vi "Core Iterate.vi"(8 "error in (no error)":errorcluster, 11 "Function in":refnum<class "Function.lvclass">) -> (0 "error out":errorcluster, 3 "Function out":refnum<class "Function.lvclass">)   [LabVIEW 2016, in "Function Actor.lvlib" / "Function.lvclass"]
uses:
  <userlib>/Common Components/Function Actor/Function.lvclass
  C:/Program Files (x86)/National Instruments/LabVIEW 2016/vi.lib/ActorFramework/Actor/Actor.lvclass
  <vilib>/ActorFramework/Actor/Actor.lvclass/Actor.ctl
  <vilib>/ActorFramework/Message Enqueuer/Message Enqueuer.lvclass/Message Enqueuer.ctl
  <userlib>/Common Components/Function Actor/Function.lvclass/Function.ctl
  <userlib>/Common Components/Function Actor/Accessors/Read polling interval (ms).vi
  <vilib>/ActorFramework/Message Enqueuer/Init from Existing Queue.vi
  <vilib>/ActorFramework/Message Enqueuer/Enqueue.vi
  <userlib>/Common Components/Function Messages/Monitoring Msg/Monitoring Msg.lvclass
  C:/Program Files (x86)/National Instruments/LabVIEW 2016/vi.lib/ActorFramework/Message/Message.lvclass
  <userlib>/Common Components/Function Messages/Updating Msg/Updating Msg.lvclass
  <userlib>/Common Components/Function Messages/Dec No of Core Iter Msg/Wait till Interval Msg.lvclass
  <userlib>/Common Components/Function Actor/Messages/Acquire Msg/Core Iterate Msg.lvclass
  <vilib>/ActorFramework/Message Priority Queue/Priority Enqueue.vi
  <vilib>/ActorFramework/Message Enqueuer/Message Enqueuer.lvclass
  <vilib>/ActorFramework/Actor/Actor.lvclass
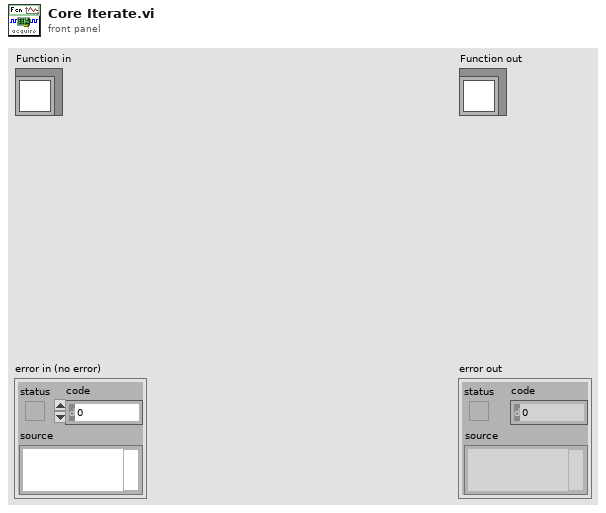
[diagram p1: front panel]
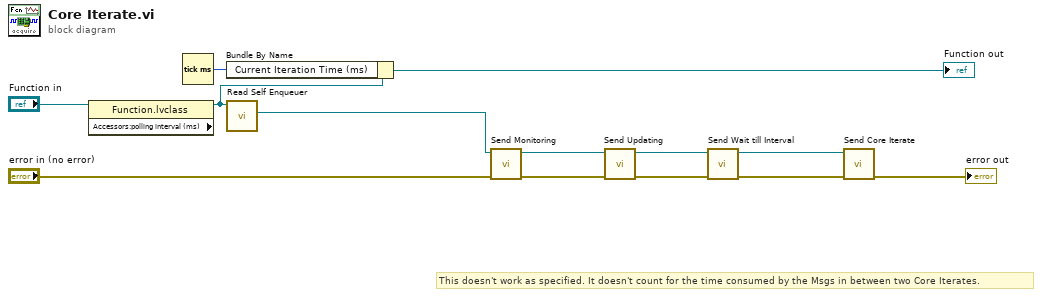
[diagram p0: block diagram]
diagram:
  # "This doesn't work as specified. It doesn't count for the time consumed by the Msgs in between two Core Iterates."
  n1 = property class="Function.lvclass" props=["Accessors:polling interval (ms)"](reference="Function in") -> (reference out=w7:refnum<class "Function.lvclass">)  [unwired: 1 in, 2 out]
  n2 = Tick Count (ms)() -> (millisecond timer value=w3:u32)
  n3 = Bundle By Name(cluster=w7, "Current Iteration Time (ms)"=w3) -> (→"Function out":refnum<class "Function.lvclass">)
  n4 = call <vilib>:"Read Self Enqueuer.vi"("Actor"=w7) -> ("Self Enqueuer"=w11:refnum<class "Message Enqueuer.lvclass">)  [unwired: 10 in]
  n5 = call <userlib>:"Send Monitoring.vi"("error in (no error)"="error in (no error)", "Message Enqueuer"=w11) -> ("error out"=w9:errorcluster, "Message Enqueuer out"=w10:refnum<class "Message Enqueuer.lvclass">)  [unwired: 8 in]
  n6 = call <userlib>:"Send Updating.vi"("error in (no error)"=w9, "Message Enqueuer"=w10) -> ("error out"=w8:errorcluster, "Message Enqueuer out"=w5:refnum<class "Message Enqueuer.lvclass">)  [unwired: 8 in]
  n7 = call <userlib>:"Send Wait till Interval.vi"("error in (no error)"=w8, "Message Enqueuer"=w5) -> ("error out"=w6:errorcluster, "Message Enqueuer out"=w1:refnum<class "Message Enqueuer.lvclass">)  [unwired: 8 in]
  n8 = call <userlib>:"Send Core Iterate.vi"("error in (no error)"=w6, "Message Enqueuer in"=w1) -> ("error out"=→"error out":errorcluster)  [unwired: 8 in, 1 out]
